vi "Variant to Type.vi"(7 "Required? (F)":bool, 10 "Type Descriptor in":T1, 11 "Variant":variant) -> (2 "Type Descriptor":T1)   [LabVIEW 2022 SP3, in "FlexBlocks Support.lvlib"]
uses:
  FlexBlocks Support.lvlib
  <vilib>/Utility/Data Type/NI_Data Type.lvlib
  Value Mode.ctl
  Terminal Direction.ctl
  Special Terminal.ctl
  Type Descriptor.ctl
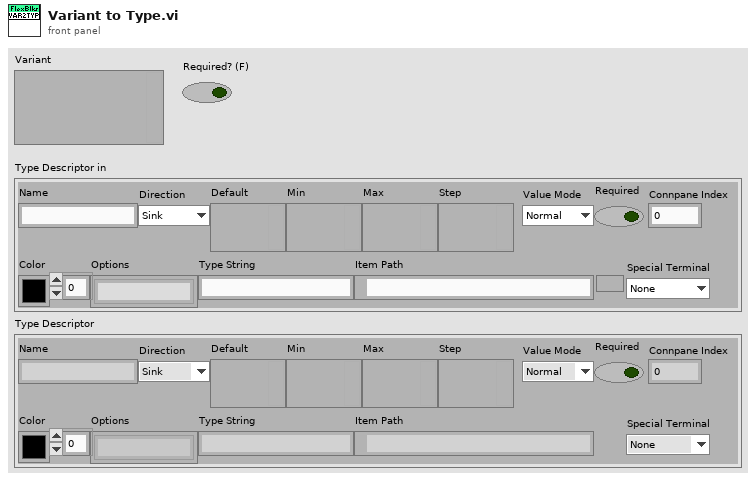
[diagram p1: front panel]
types:
  T1 = typedef "FlexBlocks Support.lvlib/Type Descriptor.ctl" = cluster{"Name":string, "Direction":T2, "Default":variant, "Min":variant, "Max":variant, "Step":variant, "Value Mode":T3, "Color":u32, "Options":string[], "Type String":string, "Item Path":path, "Required":bool, "Connpane Index":i32, "Special Terminal":T4}
  T2 = typedef "FlexBlocks Support.lvlib/Terminal Direction.ctl" = enum16{"Sink", "Source"}
  T3 = typedef "FlexBlocks Support.lvlib/Value Mode.ctl" = enum16{"Normal", "Range", "Select"}
  T4 = typedef "FlexBlocks Support.lvlib/Special Terminal.ctl" = enum16{"None", "Action", "Init", "Tag", "State in", "State out", "Error"}
  T5 = typedef "NI_Data Type.lvlib/Data Type.ctl" = enum8{"Invalid Type", "Void", "I8", "I16", "I32", "I64", "U8", "U16", "U32", "U64", "Single Float", "Double Float", "Extended Float", "Single Complex", "Double Complex", "Extended Complex", "Enum U8", "Enum U16", "Enum U32", "Enum U64", "Single Float With Unit", "Double Float With Unit", "Extended Float With Unit", "Single Complex with Unit", "Double Complex with Unit", "Extended Complex with Unit", "Boolean", "String", "Path", "Picture", "Tag", "Array", "Cluster", "Variant", "LV Variant", "Waveform", "Timestamp", "Digital Waveform", "Digital Data", "ExpressData", "Refnum", "External Data", "VI", "Poly VI", "LabVIEW Class Instance", "Fixed Point", "Set Collection", "Map Collection"}
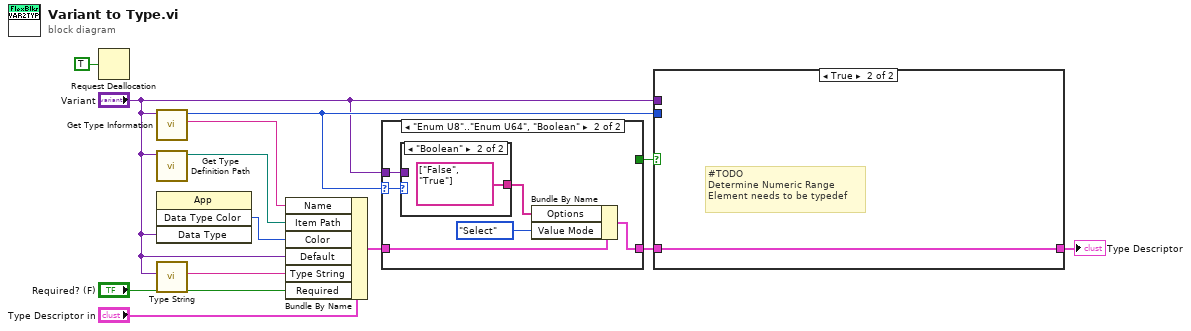
[diagram p0: block diagram]
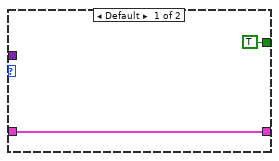
[diagram p2: hidden frame]
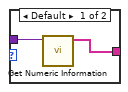
[diagram p3: hidden frame]
diagram:
  n1 = Request Deallocation(TRUE ("flag")) -> ()
  n2 = call <vilib>:"Get Type Information.vi"("variant"="Variant") -> ("name"=w7:string, "type"=w5:T5)  [unwired: 6 in, 3 out]
  n3 = call <vilib>:"Get Type Definition Path.vi"("variant"="Variant") -> ("type definition path"=w8:path)  [unwired: 9 in, 1 out]
  n4 = invoke class="App" method="Data Type Color"("Data Type"="Variant") -> ("Data Type Color"=w9:u32)  [unwired: 3 in, 3 out]
  n5 = call "Type String.vi"("Variant"="Variant") -> ("Type String"=w10:string)  [unwired: 10 in]
  n6 = Bundle By Name(cluster="Type Descriptor in", "Name"=w7, "Item Path"=w8, "Color"=w9, "Default"="Variant", "Type String"=w10, "Required"="Required? (F)") -> (w6:T1)
  n7 = case shown="\"Enum U8\"..\"Enum U64\", \"Boolean\"" w5 {
    selector: w5 -> [_ w21]
    tunnel: w6 -> [w15 w19]
    tunnel: "Variant" -> [_ w20]
    tunnel: [w15 w16] -> w3
    tunnel: [TRUE _] -> w2
    frame Default {
    }
    frame "Enum U8".."Enum U64", "Boolean" {
      n8 = case shown="\"Boolean\"" w21 {
        tunnel: w20 -> [w23 _]
        tunnel: [w22 string[] ["False", "True"]] -> w17
        frame Default {
          n9 = call <vilib>:"Get Numeric Information.vi"("variant"=w23) -> ("enum names"=w22:string[])  [unwired: 7 in, 3 out]
        }
        frame "Boolean" {
        }
      }
      n10 = Bundle By Name(cluster=w19, "Options"=w17, "Value Mode"=Value_Mode."Select") -> (w16:T1)
    }
  }
  n11 = case shown="True" w2 {
    tunnel: "Variant" -> [_ _]
    tunnel: w5 -> [_ _]
    tunnel: w3 -> [w25 w26]
    tunnel: [w25 w26] -> w1
    frame False {
    }
    frame True {
      # "#TODO\nDetermine Numeric Range\nElement needs to be typedef"
    }
  }
  "Type Descriptor" <- w1
